vi "Test Scaler Data to Wave.vi"(7 "Datatype":string, 8 "error in (no error)":errorcluster, 9 "Data":variant, 10 "Dimension":string, 11 "Flag":string) -> (0 "error out":errorcluster)   [LabVIEW 2019, in "LV-Data.ITX.lvclass"]
uses:
  LV-Data.ITX.lvclass
  <vilib>/addons/_JKI Toolkits/Caraya/classes/Assert/Assert Almost Equal_Float.vi
  <vilib>/addons/_JKI Toolkits/Caraya/classes/Assert/Assert Equal Value_Variant.vi
  <vilib>/addons/_JKI Toolkits/Caraya/classes/Assert/Assert.lvclass
  <vilib>/addons/_JKI Toolkits/Caraya/classes/Test/Test.lvclass
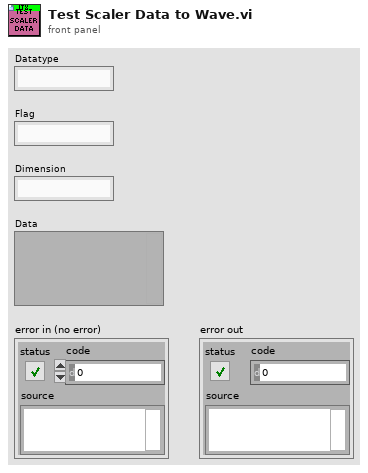
[diagram p1: front panel]
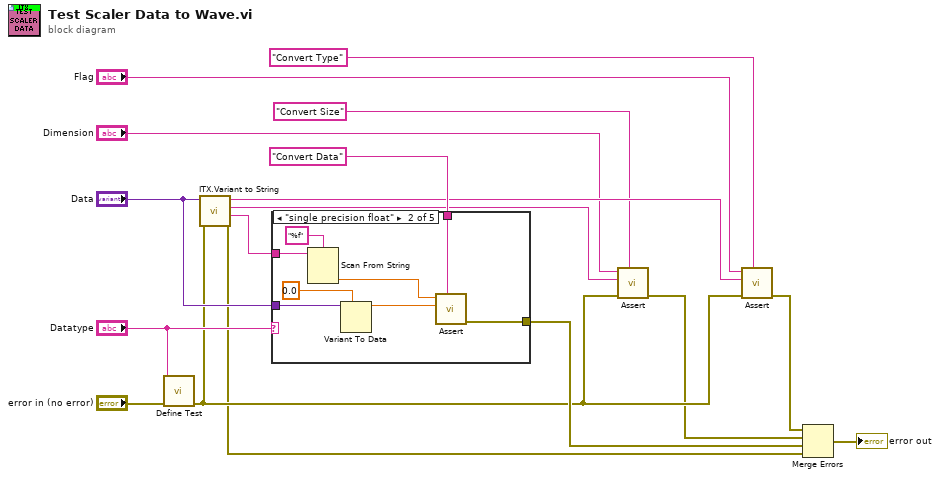
[diagram p0: block diagram]
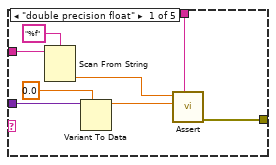
[diagram p2: hidden frame]
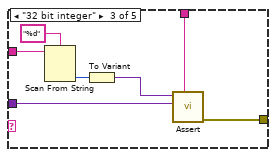
[diagram p3: hidden frame]
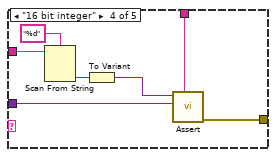
[diagram p4: hidden frame]
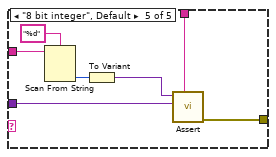
[diagram p5: hidden frame]
diagram:
  n1 = call <vilib>:"Define Test.vi"("error in (no error)"="error in (no error)", "Label (VI Title)"="Datatype") -> ("error out"=w13:errorcluster)  [unwired: 9 in]
  n2 = call "ITX.Variant to String.vi"("error in (no error)"=w13, "Data (Variant)"="Data") -> ("error out"=w11:errorcluster, "Data"=w7:string, "Size"=w3:string, "Type"=w6:string)  [unwired: 6 in]
  n3 = case shown="\"single precision float\"" "Datatype" {
    tunnel: w7 -> [w24 w32 w39 w46 w53]
    tunnel: "Data" -> [w20 w31 w36 w42 w49]
    tunnel: [w23 w27 w35 w44 w51] -> w16
    tunnel: "Convert Data" ("Label") -> [w18 w26 w34 w41 w48]
    frame "double precision float" {
      n4 = Scan From String(format string="%f", input string=w24) -> (output 1=w22:dbl)  [unwired: 3 in, 3 out]
      n5 = Variant To Data(type=0.0 ("single precision float"), Variant=w20) -> (data=w19:dbl)  [unwired: 1 in, 1 out]
      n6 = call-poly <vilib>:"Assert.vi"("Label"=w18, "Y"=w19, "X"=w22) -> ("error out"=w23:errorcluster)  [unwired: 8 in]
    }
    frame "single precision float" {
      n7 = Scan From String(format string="%f", input string=w32) -> (output 1=w28:dbl)  [unwired: 3 in, 3 out]
      n8 = Variant To Data(type=sgl 0.0 ("single precision float"), Variant=w31) -> (data=w29:sgl)  [unwired: 1 in, 1 out]
      n9 = call-poly <vilib>:"Assert.vi"("Label"=w26, "Y"=w29, "X"=w28) -> ("error out"=w27:errorcluster)  [unwired: 8 in]
    }
    frame "32 bit integer" {
      n10 = Scan From String(format string="%d", input string=w39) -> (output 1=w38:i32)  [unwired: 3 in, 3 out]
      n11 = To Variant(anything=w38) -> (Variant=w37:variant)
      n12 = call-poly <vilib>:"Assert.vi"("Label"=w34, "Y"=w36, "X"=w37) -> ("error out"=w35:errorcluster)  [unwired: 8 in]
    }
    frame "16 bit integer" {
      n13 = Scan From String(format string="%d", input string=w46) -> (output 1=w45:i32)  [unwired: 3 in, 3 out]
      n14 = To Variant(anything=w45) -> (Variant=w43:variant)
      n15 = call-poly <vilib>:"Assert.vi"("Label"=w41, "Y"=w42, "X"=w43) -> ("error out"=w44:errorcluster)  [unwired: 8 in]
    }
    frame "8 bit integer", Default {
      n16 = Scan From String(format string="%d", input string=w53) -> (output 1=w52:i32)  [unwired: 3 in, 3 out]
      n17 = To Variant(anything=w52) -> (Variant=w50:variant)
      n18 = call-poly <vilib>:"Assert.vi"("Label"=w48, "Y"=w49, "X"=w50) -> ("error out"=w51:errorcluster)  [unwired: 8 in]
    }
  }
  n19 = call-poly <vilib>:"Assert.vi"("Label"="Convert Size", "error in (no error)"=w13, "Y"=w3, "X"="Dimension") -> ("error out"=w9:errorcluster)  [unwired: 7 in]
  n20 = call-poly <vilib>:"Assert.vi"("Label"="Convert Type", "error in (no error)"=w13, "Y"=w6, "X"="Flag") -> ("error out"=w8:errorcluster)  [unwired: 7 in]
  n21 = Merge Errors(w8, w9, w16, w11) -> (→"error out":errorcluster)
